vi "Real-Time Main.vi"() -> ()   [LabVIEW 2016]
uses:
  <vilib>/userdefined/High Color/IMAQdx.ctl
  <vilib>/Platform/TimedLoop/XDataNode/timing_clust.ctl
  <vilib>/Platform/TimedLoop/XDataNode/nitl_modes.ctl
  <vilib>/Platform/TimedLoop/XDataNode/wakeup.ctl
  <vilib>/Platform/TimedLoop/XDataNode/XDataNode.xnode
  <vilib>/Platform/TimedLoop/XDataNode/XDNodeRunTimeDep.lvlib
  <vilib>/vision/driver/NI_Vision_Acquisition_Software.lvlib
panel:
  out "Image Pixels (U32) 2":u32[][](array[numeric])
  out "# elements read":u32
  out "# elements write":u32
  out "Image Pixels (U32)":u32[](array[numeric])
  out "Image":T1(plugin-control)
  out "error out":errorcluster
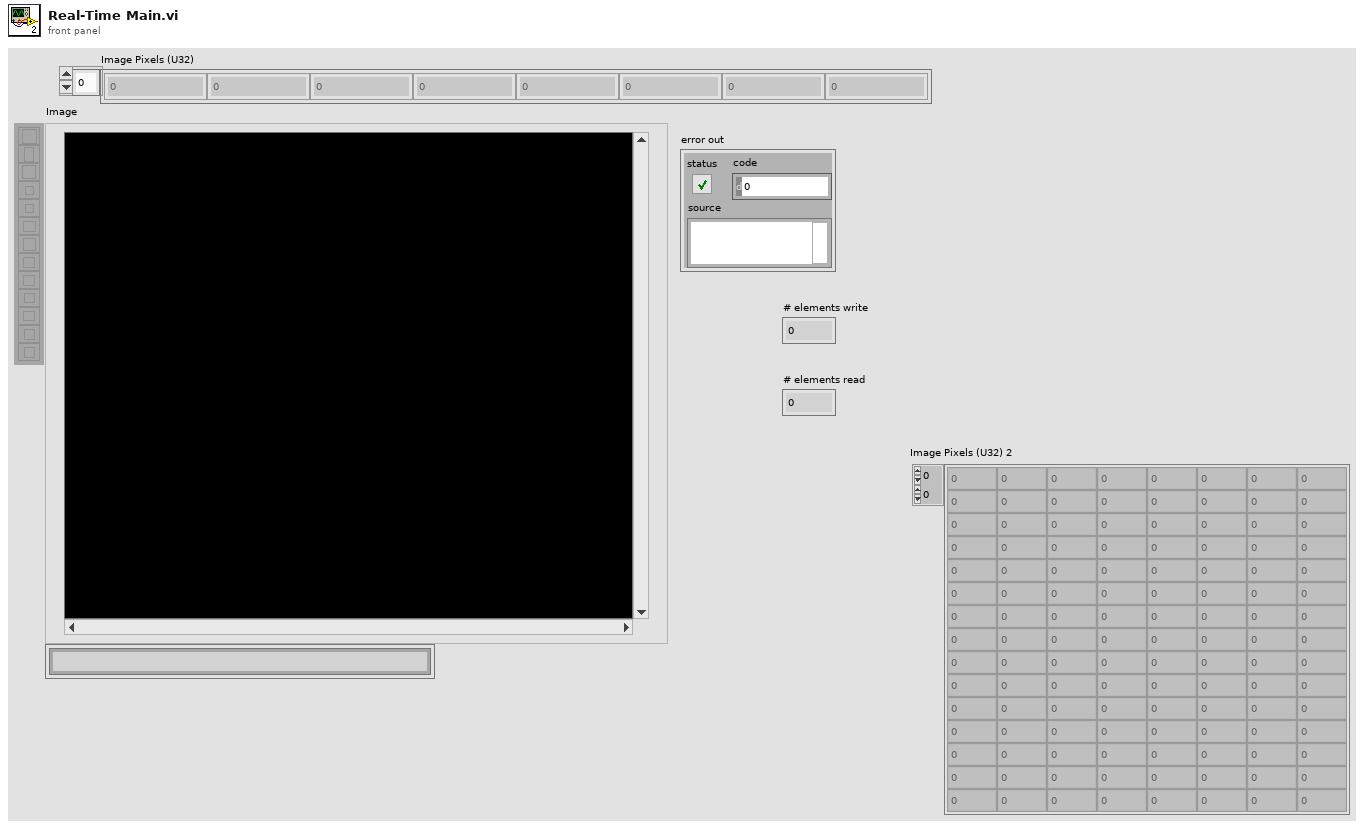
[diagram p1: front panel]
types:
  T1 = typedef "IMAQ Image.ctl" = refnum<image>
  T2 = typedef "IMAQdx.ctl" = refnum<k21>
  T3 = typedef "XDNodeRunTimeDep.lvlib/timing_clust.ctl" = cluster{"Expected End [f-1]":u64, "Actual End [f-1]":u64, "Finished Late? [f-1]":bool, "Expected End [i-1]":u64, "Actual End [i-1]":u64, "Finished Late? [i-1]":bool, "Expected Start [i]":u64, "Actual Start [i]":u64, "Expected Start [f]":u64, "Actual Start [f]":u64, "Source Name":string, "Structure Name":string, "Period":i64, "Deadline":i64, "Offset":i64, "Start":i64, "Priority":i32, "Timeout":i32, "Mode":T4, "Wakeup Reason":T5, "Error":errorcluster, "Source Type":string, "Secondary Source Type":string, "Global End Time":u64, "Global Start Time":u64, "Frame Duration":u64, "Iteration Duration":u64, "Assigned CPU":i32, "I/O Scan Engine Mode":u32}
  T4 = typedef "XDNodeRunTimeDep.lvlib/nitl_modes.ctl" = enum32{"No Change", "Process missed periods, maintain original phase", "Discard missed periods, maintain original phase", "Process missed periods, ignore original phase", "Discard missed periods, ignore original phase"}
  T5 = typedef "XDNodeRunTimeDep.lvlib/wakeup.ctl" = enum32{"Normal", "Aborted", "Asynchronous wakeup", "Timing source error", "Timed loop error", "Timeout"}
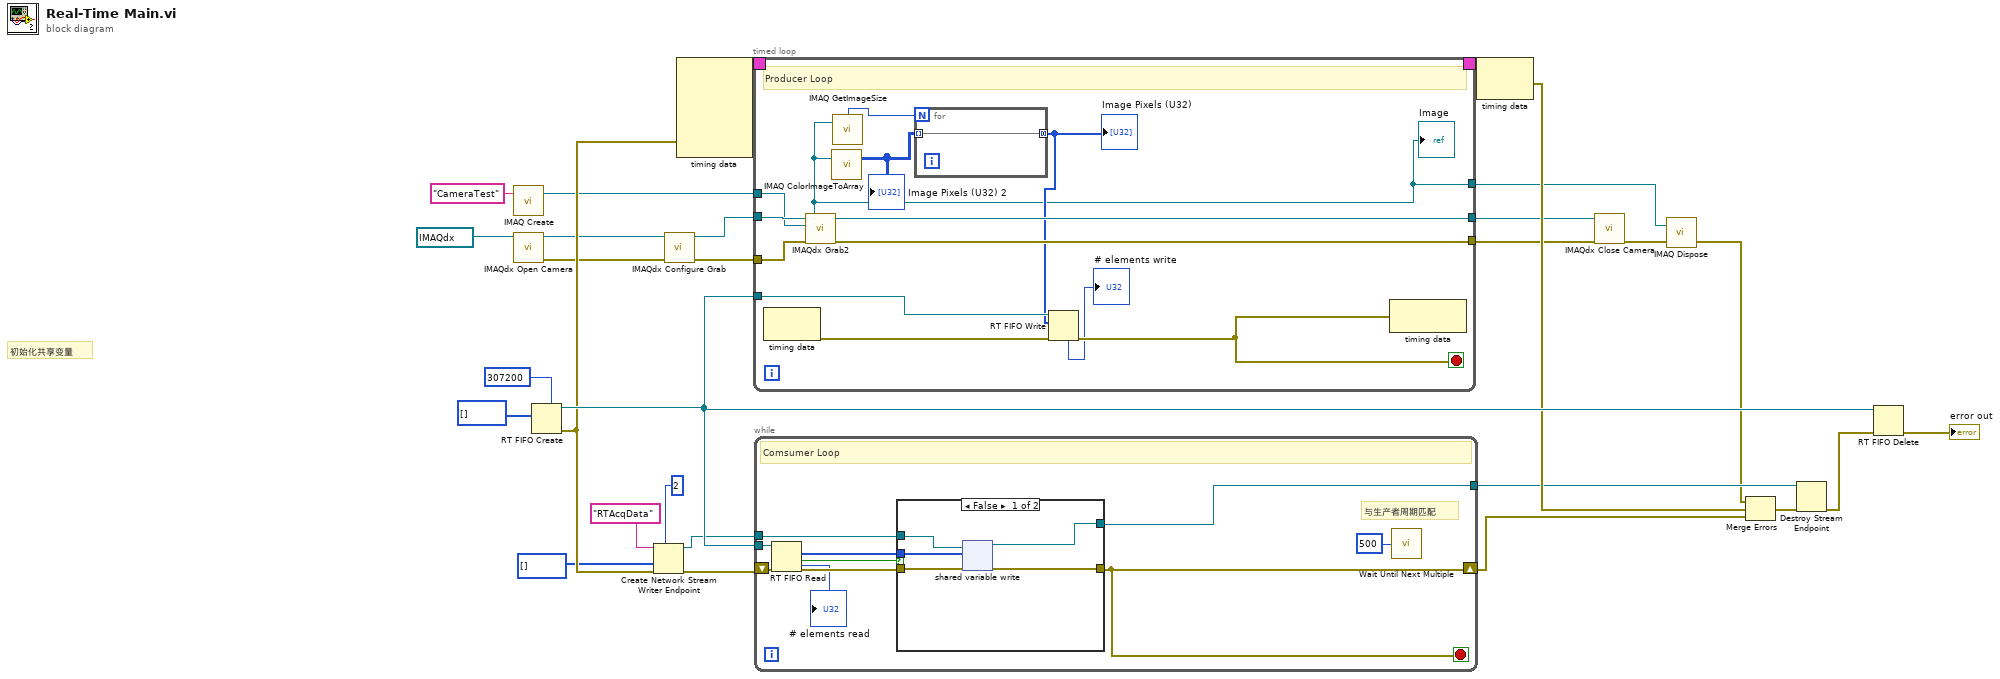
[diagram p0: block diagram]
diagram:
  # "初始化共享变量"
  n1 = call "IMAQ Create"("Image Name"="CameraTest") -> ("New Image"=w11:T1)  [unwired: 4 in, 1 out]
  n2 = call <vilib>:"IMAQdx Open Camera.vi"("Session In"=T2 "cam0") -> ("error out"=w15:errorcluster, "Session Out"=w14:T2)  [unwired: 9 in]
  n3 = RT FIFO Create(1:i32[] [], 6:u32 307200 ("elements in array (1)")) -> (8:w26:refnum<k33>, 11:w21:errorcluster)  [unwired: 6 in, 1 out]
  n4 = Create Network Stream Writer Endpoint(7:2 ("writer buffer size"), 8:w21, 9:i32[] [], 11:"RTAcqData" ("writer name")) -> (0:w20:errorcluster, 3:w19:refnum<k21>)  [unwired: 3 in]
  n5 = call <vilib>:"IMAQdx Configure Grab.vi"("error in"=w15, "Session In"=w14) -> ("error out"=w13:errorcluster, "Session Out"=w12:T2)  [unwired: 8 in]
  n6 = node-c288(w21) -> (w29:T3)  [unwired: 4 in]
  n7 = timed-loop {
    timing: w29 -> [_]
    timing-out: [_] -> w28
    tunnel: w26 -> [w40]
    tunnel: w13 -> [w39]
    tunnel: w12 -> [w38]
    tunnel: w11 -> [w37]
    tunnel: [w36] -> w10
    tunnel: [w31] -> w8
    tunnel: [w35] -> w7
    stop <- w41 stop-if-true
    # "Producer Loop"
    n8 = node-c288() -> (w42:errorcluster)  [unwired: 1 in]
    n9 = call <vilib>:"IMAQdx Grab2.vi"("error in"=w39, "Image In"=w37, "Session In"=w38) -> ("error out"=w35:errorcluster, "Image Out"=w31:T1, "Session Out"=w36:T2)  [unwired: 5 in, 1 out]
    "Image" <- w31
    n10 = call "IMAQ ColorImageToArray"("Image"=w31) -> ("Image Pixels (U32)"=w33:u32[][])  [unwired: 3 in, 2 out]
    "Image Pixels (U32) 2" <- w33
    n11 = call "IMAQ GetImageSize"("Image"=w31) -> ("X Resolution"=w34:i32)  [unwired: 3 in, 2 out]
    n12 = for {
      N: w34 -> [_]
      tunnel: w33 -> [w43] mode=indexing
      tunnel: [w43] -> w32 mode=concatenating
    }
    "Image Pixels (U32)" <- w32
    n13 = RT FIFO Write(0:w40, 1:w32, 3:w42) -> (7:→"# elements write":u32, 11:w41:errorcluster)  [unwired: 2 in, 2 out]
    n14 = node-c288(w41) -> ()  [unwired: 1 out]
  }
  n15 = while {
    tunnel: w26 -> [w57]
    shift-right: [w52] -> w24
    shift-left: w20 -> [w56]
    tunnel: w19 -> [w51]
    tunnel: [w50] -> w16
    stop <- w52 stop-if-true
    # "与生产者周期匹配"
    # "Comsumer Loop"
    n16 = RT FIFO Read(0:w57, 3:w56) -> (7:→"# elements read":u32, 9:w54:i32[], 10:w55:bool, 11:w53:errorcluster)  [unwired: 2 in, 1 out]
    n17 = case shown="False" w55 {
      tunnel: w54 -> [w59 _]
      tunnel: w53 -> [w62 w65]
      tunnel: [w61 w65] -> w52
      tunnel: w51 -> [w63 w64]
      tunnel: [w60 w64] -> w50
      frame False {
        n18 = shared-variable-write(w63, w62, w59) -> (w60:refnum<k21>, w61:errorcluster)  [unwired: 1 in, 1 out]
      }
      frame True {
      }
    }
    n19 = call "Wait Until Next Multiple"("Count(mSec)"=u32 500) -> ()  [unwired: 1 out]
  }
  n20 = node-c288(w28) -> (w25:errorcluster)
  n21 = call <vilib>:"IMAQdx Close Camera.vi"("error in"=w7, "Session In"=w10) -> ("error out"=w9:errorcluster)  [unwired: 9 in]
  n22 = call "IMAQ Dispose"("Image"=w8, "error in (no error)"=w9) -> ("error out"=w6:errorcluster)  [unwired: 4 in]
  n23 = Merge Errors(w6, w25, w24) -> (w18:errorcluster)
  n24 = Destroy Stream Endpoint(8:w18, 11:w16) -> (0:w17:errorcluster)
  n25 = RT FIFO Delete(0:w26, 3:w17) -> (11:→"error out":errorcluster)  [unwired: 1 in]
